vi "MakeChannelColorArray.vi"(2 "ArrayLength":u32, 3 "FalseColorDat":cluster{dbl, dbl}[](array[cluster])) -> (1 "GradualChangeColorBar1DArray":u8[](array[numeric]))   [LabVIEW 2016]
panel:
  # "0~1"
  # "0~255,Z+"
  # "0~1"
  # ">0"
  # "根据伪彩色折点数据生成一定长度的渐变条的一维RGB数据数组"
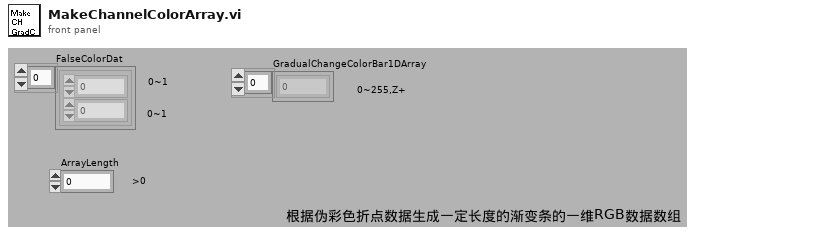
[diagram p1: front panel]
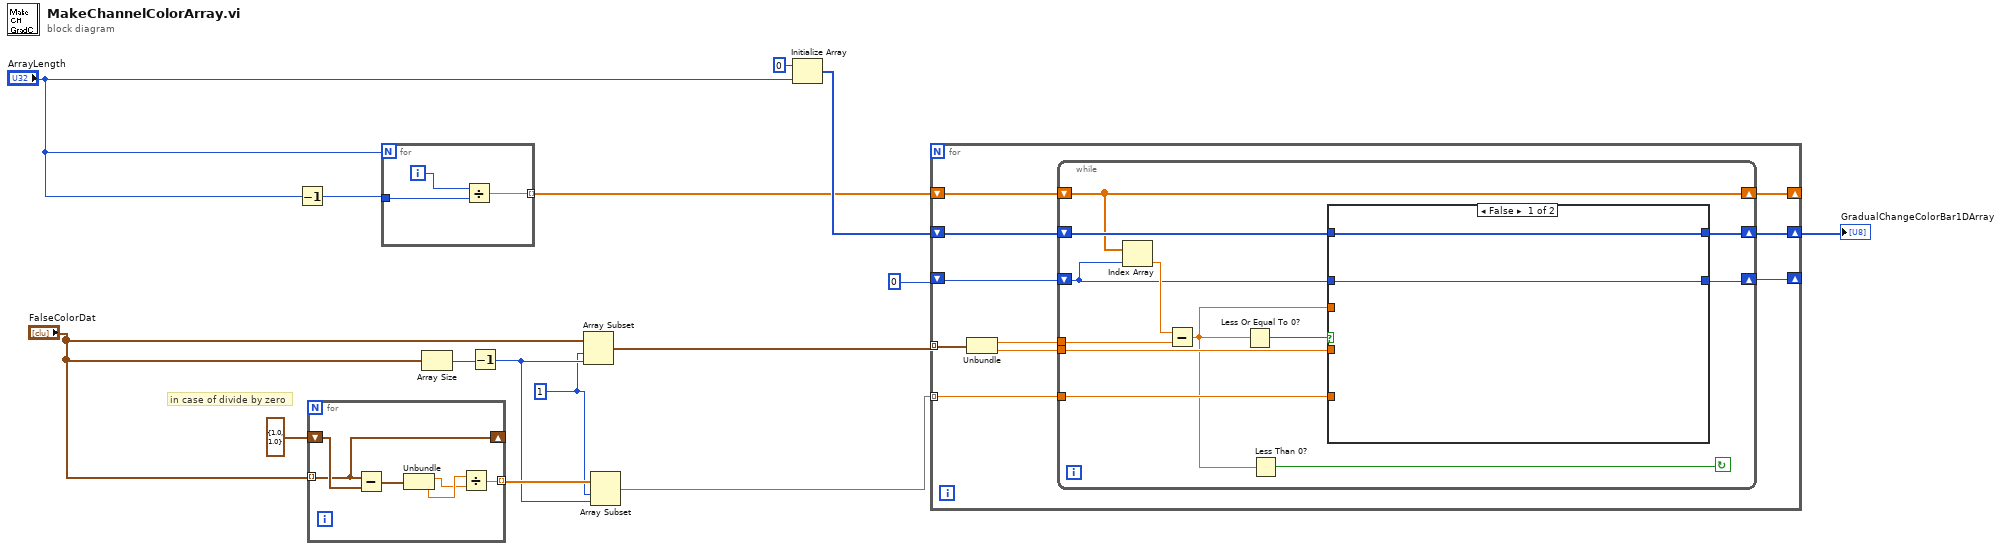
[diagram p0: block diagram]
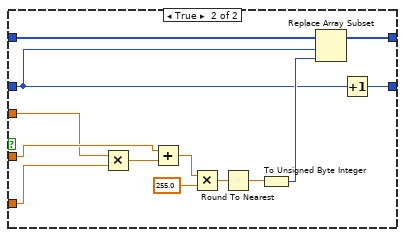
[diagram p2: hidden frame]
diagram:
  w1 = 1 ("索引")
  # "in case of divide by zero"
  n1 = Decrement(x="ArrayLength") -> (x-1=w9:u32)
  n2 = for {
    tunnel: "FalseColorDat" -> [w20] mode=indexing
    shift-right: [w20] -> _
    shift-left: cluster{dbl, dbl} {1.0, 1.0} -> [w21]
    tunnel: [w16] -> w7 mode=indexing
    n3 = Subtract(x=w20, y=w21) -> (x-y=w19:cluster{dbl, dbl})
    n4 = Unbundle(w19) -> (w17:dbl, w18:dbl)
    n5 = Divide(x=w18, y=w17) -> (x/y=w16:dbl)
  }
  n6 = for {
    N: "ArrayLength" -> [_]
    tunnel: w9 -> [w23]
    tunnel: [w22] -> w5 mode=indexing
    i -> [w24]
    n7 = Divide(x=w24, y=w23) -> (x/y=w22:dbl)
  }
  n8 = Array Size(array="FalseColorDat") -> (size(s)=w12:i32)
  n9 = Decrement(x=w12) -> (x-1=w2:i32)
  n10 = Array Subset(array="FalseColorDat", index=w1, length=w2) -> (w3:cluster{dbl, dbl}[])
  n11 = Array Subset(array=w7, index=w1, length=w2) -> (w8:dbl[])
  n12 = Initialize Array(u8 0 ("索引"), "ArrayLength") -> (w13:u8[])
  n13 = for {
    shift-right: [w29] -> _
    shift-left: 0 ("索引") -> [w33]
    tunnel: w8 -> [w32] mode=indexing
    shift-right: [w30] -> w11
    shift-left: w13 -> [w31]
    shift-right: [w28] -> _
    shift-left: w5 -> [w34]
    tunnel: w3 -> [w27] mode=indexing
    n14 = Unbundle(w27) -> (w26:dbl, w25:dbl)
    n15 = while {
      shift-right: [w38] -> w29
      shift-left: w33 -> [w40]
      tunnel: w26 -> [w42]
      tunnel: w25 -> [w45]
      tunnel: w32 -> [w46]
      shift-right: [w39] -> w30
      shift-left: w31 -> [w41]
      shift-right: [w35] -> w28
      shift-left: w34 -> [w35]
      stop <- w36 continue-if-true
      n16 = Index Array(array=w35, index=w40) -> (element=w43:dbl)
      n17 = Subtract(x=w43, y=w42) -> (x-y=w44:dbl)
      n18 = Less Or Equal To 0?(x=w44) -> (x <= 0?=w37:bool)
      n19 = Less Than 0?(x=w44) -> (x < 0?=w36:bool)
      n20 = case shown="False" w37 {
        tunnel: w46 -> [_ w61]
        tunnel: [w48 w51] -> w39
        tunnel: w45 -> [_ w58]
        tunnel: w44 -> [_ w54]
        tunnel: w41 -> [w48 w53]
        tunnel: w40 -> [w47 w50]
        tunnel: [w47 w49] -> w38
        frame False {
        }
        frame True {
          n21 = Multiply(x=w54, y=w61) -> (x*y=w60:dbl)
          n22 = Add(x=w58, y=w60) -> (x+y=w56:dbl)
          n23 = Multiply(x=w56, y=255.0) -> (x*y=w55:dbl)
          n24 = Round To Nearest(number=w55) -> (nearest integer value=w59:dbl)
          n25 = To Unsigned Byte Integer(number=w59) -> (unsigned 8bit integer=w52:u8)
          n26 = Replace Array Subset(array=w53, new element=w52, index=w50) -> (w51:u8[])
          n27 = Increment(x=w50) -> (x+1=w49:i32)
        }
      }
    }
  }
  "GradualChangeColorBar1DArray" <- w11
